vi "insert_node.vi"(8 "error in (no error)":errorcluster, 9 "node":refnum<class "Node.lvclass">, 11 "graph":refnum<class "Graph.lvclass">) -> (0 "error out":errorcluster, 1 "node unchanged?":bool, 2 "node already included?":bool, 3 "graph out":refnum<class "Graph.lvclass">)   [LabVIEW 2020, in "graph.lvlib" / "Graph.lvclass"]
uses:
  Graph.lvclass
  Node/Node.lvclass
  Graph.lvclass/Graph.ctl
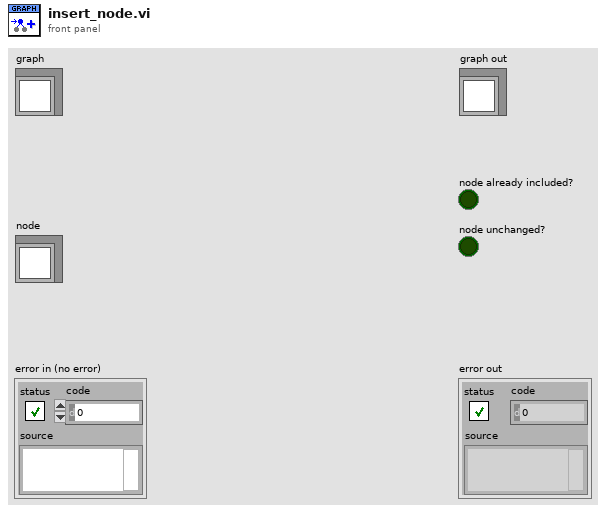
[diagram p1: front panel]
types:
  T1 = map{refnum<class "ID.lvclass">, refnum<class "Node.lvclass">}
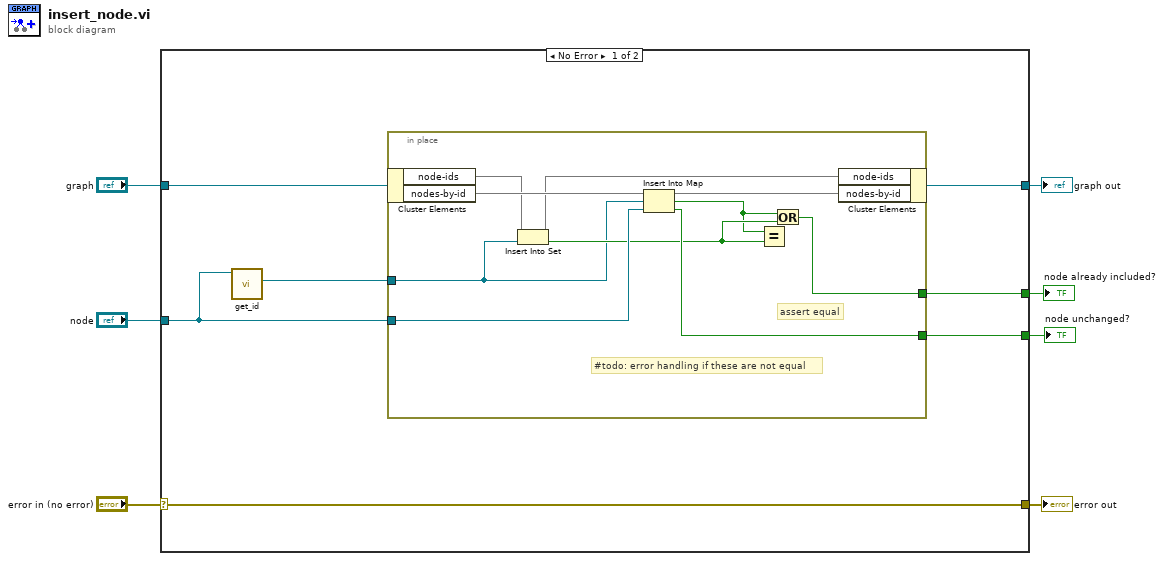
[diagram p0: block diagram]
diagram:
  n1 = case shown="No Error" "error in (no error)" {
    selector: "error in (no error)" -> [w10 w26]
    tunnel: [w10 w26] -> w6
    tunnel: [w13 w25] -> w4
    tunnel: "graph" -> [w14 w25]
    tunnel: "node" -> [w12 _]
    tunnel: [w11 _] -> w2
    tunnel: [w9 _] -> w1
    frame No Error {
      n2 = call "get_id.vi"("node"=w12) -> ("node-id"=w8:refnum<class "ID.lvclass">)  [unwired: 10 in]
      n3 = in-place {
        in-place-border: w8 -> [w15]
        in-place-border: w12 -> [w23]
        in-place-border: [w21] -> w11
        in-place-border: [w16] -> w9
        # "assert equal"
        # "#todo: error handling if these are not equal"
        n4 = in-place-cluster #1(w14) -> ("node-ids"=w20:set{refnum<class "ID.lvclass">}, "nodes-by-id"=w24:T1)
        n5 = Insert Into Set(10:w15, 11:w20) -> (2:w18:bool, 3:w19:set{refnum<class "ID.lvclass">})
        n6 = Insert Into Map(map in=w24, key=w15, value=w23) -> (map out=w22:T1, key already included?=w17:bool, value unchanged?=w21:bool)
        n7 = Equal?(x=w17, y=w18) -> ()  [unwired: 1 out]
        n8 = Or(x=w17, y=w18) -> (x .or. y?=w16:bool)
        n9 = in-place-cluster #1("node-ids"=w19, "nodes-by-id"=w22) -> (w13:refnum<class "Graph.lvclass">)
      }
    }
    frame Error {
    }
  }
  "error out" <- w6
  "graph out" <- w4
  "node unchanged?" <- w2
  "node already included?" <- w1
